vi "Read Results from processing.vi"(8 "error in":errorcluster, 11 "BuckBoost runtime in":refnum<class "BuckBoost runtime.lvclass">) -> (0 "error out":errorcluster, 2 "Results from processing":T1, 3 "BuckBoost runtime out":refnum<class "BuckBoost runtime.lvclass">)   [LabVIEW 2017, in "BuckBoost runtime.lvclass"]
uses:
  BuckBoost runtime.lvclass
  configuration/result data indices.ctl
  BuckBoost runtime.lvclass/BuckBoost runtime.ctl
  configuration/BuckBoost configuration.lvclass
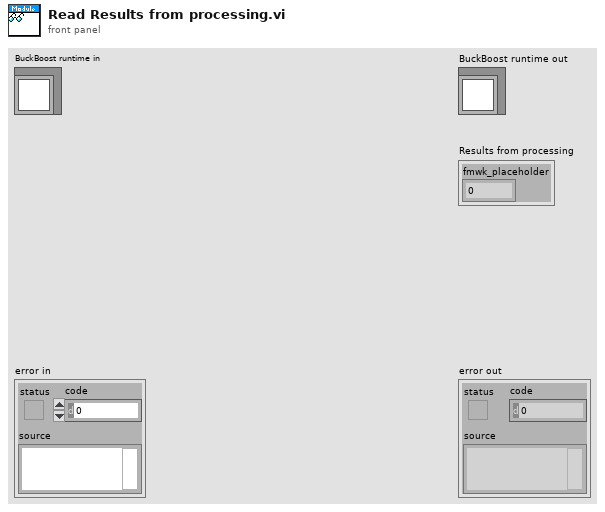
[diagram p1: front panel]
types:
  T1 = typedef "BuckBoost configuration.lvclass/result data indices.ctl" = cluster{"fmwk_placeholder":i32}
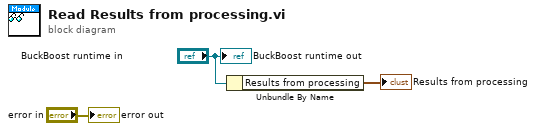
[diagram p0: block diagram]
diagram:
  n1 = Unbundle By Name("BuckBoost runtime in") -> ("Results from processing"=→"Results from processing":T1)
  "error out" <- "error in"
  "BuckBoost runtime out" <- "BuckBoost runtime in"
